vi "svx_Timebase X FString Write.vi"(4 "error in (no error)":errorcluster, 5 "Value":string, 6 "Container State":T5, 7 "Display State In":T1={"X Scale"={"Name"="Time", "FString"="%#.2g", "Major Color"=16777238, "Minor Color"=16777216, "Grid Style"=1, "Maximum"=0.5, "Minimum"=0.0, "Autoscale"=TRUE, "Show Scale Label"={"Probe X"=FALSE, "Probe Y"=TRUE}, "Show Scale"={"Probe X"=TRUE, "Probe Y"=TRUE}, "Autoscale Once"=FALSE}, "Y Scale"={"Name"="Amplitude", "FString"="%#.2g", "Major Color"=16777238, "Minor Color"=16777216, "Scale Visible"=TRUE, " Label Visible"=TRUE, "Grid Style"=1, "Autoscale"=TRUE, "Maximum"={"Probe X"=1.0, "Probe Y"=1.0}, "Minimum"={"Probe X"=-1.0, "Probe Y"=-1.0}, "Autoscale Once"=FALSE}, "Plot"={"Point Style"=0, "Line Width"=0, "Line Style"=0, "Plot Color"=16860, "Point/fill"=16860}, "Tacho Point Color"=16711680, "Property Name"=[], "Container Bounds"={"Width"=640, "Height"=360}, "Background color"=16777226, "Legend Visible"=TRUE, "Scale Range Change"=refnum, "Strings[]"={"Custom pair name"=FALSE, "Row Strings []"=[], "Column Strings []"=[]}, "Cursor"={"Cursor Point Style"=13, "Cursor Style"=5, "Cursor Line Width"=1, "Cursor Line Style"=0, "Cursor Color"=16860, "Cursor Name Visible"=TRUE, "Cursor Visible"=TRUE, "Cursor Lock"=FALSE, "Cursor Index"=0}, "Index"=[], "Legend Width"=200, " Parents Tags"=[], "Children Tags"=[], "Open?"=[], "Label"="Timebase Plot", "Cursor X Pos"={"X"=0.0, "Y"=0.0}, "Cursor Y Pos"={"X"=0.0, "Y"=0.0}, "Graph Type"=enum."Probe X and Y", "Prev Graph Type"=enum."Probe X and Y", "Prev Legend Visible"=TRUE, "Cursor Release"=refnum, "Pair Strings Changed?"=FALSE, "Cursor ID"=refnum, "Legend Background"=16777226, "Legend Font"=16777222, "Probe Y Label"="Probe Y", "Probe X Label"="Probe X", "Probe X Label Visible"=TRUE, "Probe Y Label Visible"=TRUE, "Tree Item Width"=200, "# Custom RowStr"=0, "# Custom ColStr"=0, "Property Name"=refnum, "Data Related State"=refnum}) -> (0 "error out":errorcluster, 3 "Display State Out":T1={"X Scale"={"Name"="Time", "FString"="%#.2g", "Major Color"=16777238, "Minor Color"=16777216, "Grid Style"=1, "Maximum"=0.5, "Minimum"=0.0, "Autoscale"=TRUE, "Show Scale Label"={"Probe X"=FALSE, "Probe Y"=TRUE}, "Show Scale"={"Probe X"=TRUE, "Probe Y"=TRUE}, "Autoscale Once"=FALSE}, "Y Scale"={"Name"="Amplitude", "FString"="%#.2g", "Major Color"=16777238, "Minor Color"=16777216, "Scale Visible"=TRUE, " Label Visible"=TRUE, "Grid Style"=1, "Autoscale"=TRUE, "Maximum"={"Probe X"=1.0, "Probe Y"=1.0}, "Minimum"={"Probe X"=-1.0, "Probe Y"=-1.0}, "Autoscale Once"=FALSE}, "Plot"={"Point Style"=0, "Line Width"=0, "Line Style"=0, "Plot Color"=16860, "Point/fill"=16860}, "Tacho Point Color"=16711680, "Property Name"=[], "Container Bounds"={"Width"=640, "Height"=360}, "Background color"=16777226, "Legend Visible"=TRUE, "Scale Range Change"=refnum, "Strings[]"={"Custom pair name"=FALSE, "Row Strings []"=[], "Column Strings []"=[]}, "Cursor"={"Cursor Point Style"=13, "Cursor Style"=5, "Cursor Line Width"=1, "Cursor Line Style"=0, "Cursor Color"=16860, "Cursor Name Visible"=TRUE, "Cursor Visible"=TRUE, "Cursor Lock"=FALSE, "Cursor Index"=0}, "Index"=[], "Legend Width"=200, " Parents Tags"=[], "Children Tags"=[], "Open?"=[], "Label"="Timebase Plot", "Cursor X Pos"={"X"=0.0, "Y"=0.0}, "Cursor Y Pos"={"X"=0.0, "Y"=0.0}, "Graph Type"=enum."Probe X and Y", "Prev Graph Type"=enum."Probe X and Y", "Prev Legend Visible"=TRUE, "Cursor Release"=refnum, "Pair Strings Changed?"=FALSE, "Cursor ID"=refnum, "Legend Background"=16777226, "Legend Font"=16777222, "Probe Y Label"="Probe Y", "Probe X Label"="Probe X", "Probe X Label Visible"=TRUE, "Probe Y Label Visible"=TRUE, "Tree Item Width"=200, "# Custom RowStr"=0, "# Custom ColStr"=0, "Property Name"=refnum, "Data Related State"=refnum})   [LabVIEW 2017, in "SVX Timebase.xctl"]
uses:
  <vilib>/addons/_XControls/Timebase Plot/SVX Timebase.xctl
  <vilib>/_xctls/Container State.ctl
  <vilib>/addons/_XControls/Timebase Plot/subVIs/svx_Timebase State.ctl
  <vilib>/addons/_XControls/Timebase Plot/subVIs/svx_Timebase Bounds.ctl
  <vilib>/addons/_XControls/Timebase Plot/subVIs/svx_Timebase Graph Types.ctl
  <vilib>/addons/_XControls/Timebase Plot/subVIs/svx_Timebase Data Related State.ctl
  <vilib>/_xctls/XControlSupport.lvlib
panel:
  # "Replace the Value Control below with a Control of desired type.\nDo not remove this Control or the others from the connector pane.\nDo not change the connector pane pattern.\nThe Value control should always be the third terminal from top on the input side in the connector pane."
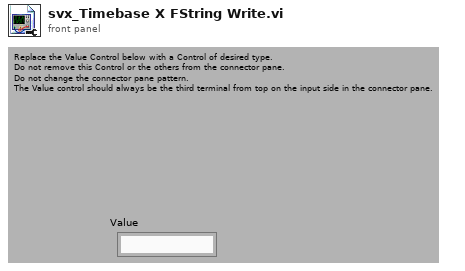
[diagram p1: front panel]
types:
  T1 = typedef "SVX Timebase.xctl/svx_Timebase State.ctl" = cluster{"X Scale":cluster{"Name":string, "FString":string, "Major Color":u32, "Minor Color":u32, "Grid Style":u16, "Maximum":dbl, "Minimum":dbl, "Autoscale":bool, "Show Scale Label":cluster{"Probe X":bool, "Probe Y":bool}, "Show Scale":cluster{"Probe X":bool, "Probe Y":bool}, "Autoscale Once":bool}, "Y Scale":cluster{"Name":string, "FString":string, "Major Color":u32, "Minor Color":u32, "Scale Visible":bool, " Label Visible":bool, "Grid Style":u16, "Autoscale":bool, "Maximum":cluster{"Probe X":dbl, "Probe Y":dbl}, "Minimum":cluster{"Probe X":dbl, "Probe Y":dbl}, "Autoscale Once":bool}, "Plot":cluster{"Point Style":u8, "Line Width":u8, "Line Style":u8, "Plot Color":u32, "Point/fill":u32}, "Tacho Point Color":u32, "Property Name":string[], "Container Bounds":T2, "Background color":u32, "Legend Visible":bool, "Scale Range Change":refnum<user-event>, "Strings[]":cluster{"Custom pair name":bool, "Row Strings []":string[], "Column Strings []":string[]}, "Cursor":cluster{"Cursor Point Style":u8, "Cursor Style":u8, "Cursor Line Width":u8, "Cursor Line Style":u8, "Cursor Color":u32, "Cursor Name Visible":bool, "Cursor Visible":bool, "Cursor Lock":bool, "Cursor Index":i32}, "Index":cluster{"Pair Index":u32, "Order Index":u32}[], "Legend Width":u32, " Parents Tags":string[], "Children Tags":string[], "Open?":bool[], "Label":string, "Cursor X Pos":cluster{"X":dbl, "Y":dbl}, "Cursor Y Pos":cluster{"X":dbl, "Y":dbl}, "Graph Type":T3, "Prev Graph Type":T3, "Prev Legend Visible":bool, "Cursor Release":refnum<user-event>, "Pair Strings Changed?":bool, "Cursor ID":refnum<k1>, "Legend Background":u32, "Legend Font":u32, "Probe Y Label":string, "Probe X Label":string, "Probe X Label Visible":bool, "Probe Y Label Visible":bool, "Tree Item Width":u32, "# Custom RowStr":u32, "# Custom ColStr":u32, "Property Name":refnum<queue>, "Data Related State":T4}
  T2 = typedef "SVX Timebase.xctl/svx_Timebase Bounds.ctl" = cluster{"Width":u32, "Height":u32}
  T3 = typedef "SVX Timebase.xctl/svx_Timebase Graph Types.ctl" = enum16{"Probe X", "Probe Y", "Probe X and Y"}
  T4 = typedef "SVX Timebase.xctl/svx_Timebase Data Related State.ctl" = refnum<queue>
  T5 = typedef "XControlSupport.lvlib/Container State.ctl" = cluster{"Indicator?":bool, "Run Mode?":bool, " Refnum":refnum<vi>}
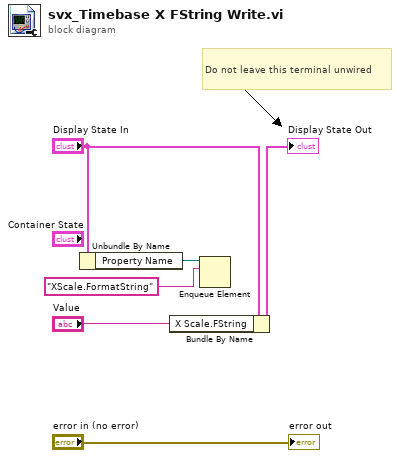
[diagram p0: block diagram]
diagram:
  # "Do not leave this terminal unwired"
  n1 = Unbundle By Name("Display State In") -> ("Property Name"=w5:refnum<queue>)
  n2 = Bundle By Name(cluster="Display State In", "X Scale.FString"="Value") -> (→"Display State Out":T1)
  n3 = Enqueue Element(queue=w5, element="XScale.FormatString" ("Property Name")) -> ()  [unwired: 2 in, 3 out]
  "error out" <- "error in (no error)"
